vi "DSF.Shared.Configuration.Get ID.vi"(11 "Configuration in":refnum<class "DSF.Shared.Configuration.lvclass">) -> (2 "id":T1, 3 "Configuration out":refnum<class "DSF.Shared.Configuration.lvclass">)   [LabVIEW 2017, in "DSF.Engine.lvlib" / "DSF.Shared.Configuration.lvclass"]
uses:
  DSF.Shared.Configuration.lvclass
  Typedefs/DSF Runtime Index.ctl
  DSF.Shared.Configuration.lvclass/DSF.Shared.Configuration.ctl
  DSF.Engine.lvlib
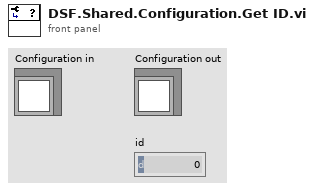
[diagram p1: front panel]
types:
  T1 = typedef "DSF.Engine.lvlib/DSF Runtime Index.ctl" = i32
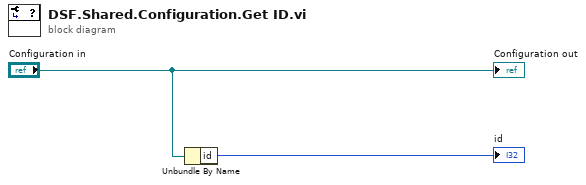
[diagram p0: block diagram]
diagram:
  n1 = Unbundle By Name("Configuration in") -> ("id"=→"id":T1)
  "Configuration out" <- "Configuration in"
